vi "SineModel.vi"(3 "output control":T1, 4 "data":variant, 5 "X":dbl[](array[numeric]), 6 "a":dbl[](array[numeric])) -> (0 "error out":errorcluster, 1 "f'(X,a)":dbl[][](array[numeric]), 2 "f(X,a)":dbl[](array[numeric]))   [LabVIEW 2015]
doc: "This template is the starting point for creating a model function to be passed to the Nonlinear Curve Fit.vi."
uses:
  <vilib>/gmath/NumericalOptimization/LM_output select.ctl
  <vilib>/gmath/NI_Gmath.lvlib
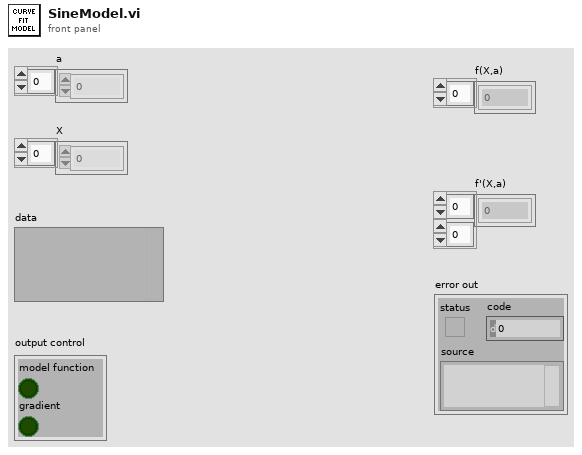
[diagram p1: front panel]
types:
  T1 = typedef "NI_Gmath.lvlib/LM_output select.ctl" = cluster{"model function":bool, "gradient":bool}
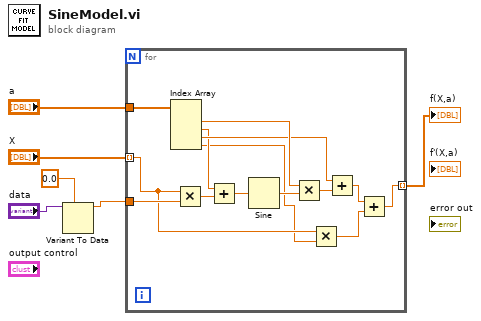
[diagram p0: block diagram]
diagram:
  n1 = Variant To Data(type=0.0, Variant="data") -> (data=w2:dbl)  [unwired: 1 in, 1 out]
  n2 = for {
    tunnel: "a" -> [w20]
    tunnel: "X" -> [w9] mode=indexing
    tunnel: w2 -> [w15]
    tunnel: [w10] -> w1 mode=indexing
    n3 = Index Array(array=w20) -> (element #1=w14:dbl, element #2=w12:dbl, element #3=w13:dbl, element #4=w8:dbl)  [unwired: 4 in]
    n4 = Multiply(x=w9, y=w15) -> (x*y=w19:dbl)
    n5 = Add(x=w12, y=w19) -> (x+y=w18:dbl)
    n6 = Sine(x=w18) -> (sin(x)=w17:dbl)
    n7 = Multiply(x=w14, y=w17) -> (x*y=w16:dbl)
    n8 = Multiply(x=w9, y=w8) -> (x*y=w7:dbl)
    n9 = Add(x=w13, y=w16) -> (x+y=w11:dbl)
    n10 = Add(x=w11, y=w7) -> (x+y=w10:dbl)
  }
  "f(X,a)" <- w1
